vi "Add New Node In XML.vi"(6 "Data":string, 8 "error in (no error)":errorcluster, 9 "Tag Name":string, 10 "DOM document":refnum<k20>, 11 "XML Project in":refnum<class "XML Project.lvclass">) -> (0 "error out":errorcluster, 3 "XML Project out":refnum<class "XML Project.lvclass">)   [LabVIEW 2015, in "XML Project.lvclass"]
uses:
  XML Project.lvclass
  <resource>/objmgr/DOMUserDefRef.rc
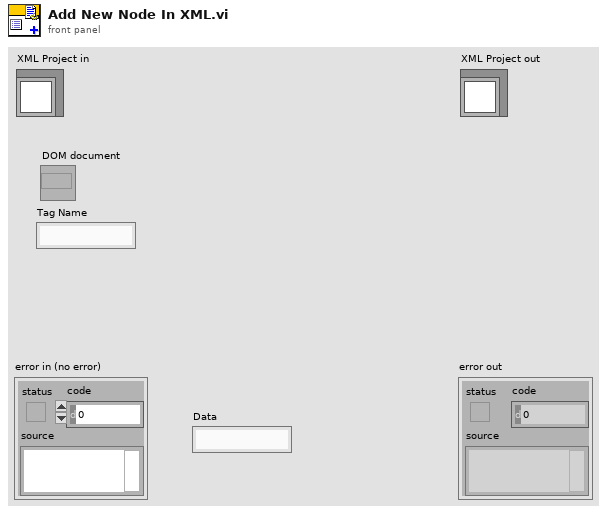
[diagram p1: front panel]
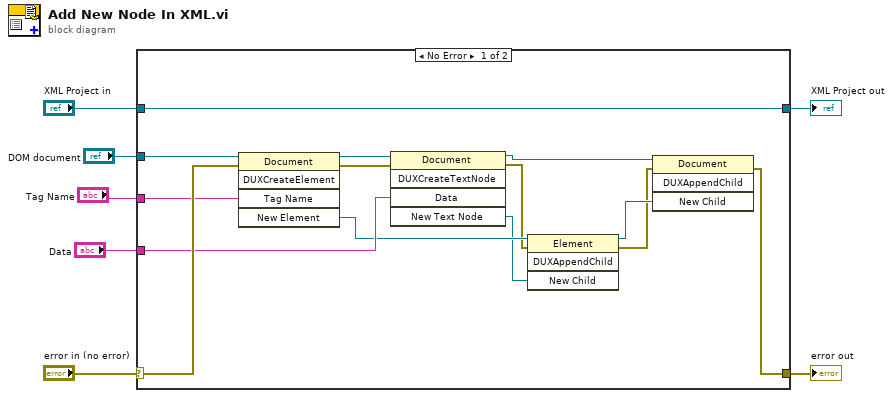
[diagram p0: block diagram]
diagram:
  n1 = case shown="No Error" "error in (no error)" {
    selector: "error in (no error)" -> [w19 w23]
    tunnel: [w8 w23] -> w6
    tunnel: [w21 w22] -> w4
    tunnel: "XML Project in" -> [w21 w22]
    tunnel: "DOM document" -> [w20 _]
    tunnel: "Tag Name" -> [w18 _]
    tunnel: "Data" -> [w15 _]
    frame No Error {
      n2 = invoke class="Document" method="DUXCreateElement"(reference=w20, error in=w19, "Tag Name"=w18) -> (reference out=w17:refnum<k20>, error out=w16:errorcluster, "New Element"=w14:refnum<k20>)  [unwired: 2 in, 2 out]
      n3 = invoke class="Document" method="DUXCreateTextNode"(reference=w17, error in=w16, "Data"=w15) -> (reference out=w11:refnum<k20>, error out=w12:errorcluster, "New Text Node"=w13:refnum<k20>)  [unwired: 2 in, 2 out]
      n4 = invoke class="Element" method="DUXAppendChild"(reference=w14, error in=w12, "New Child"=w13) -> (reference out=w10:refnum<k20>, error out=w9:errorcluster)  [unwired: 1 in, 2 out]
      n5 = invoke class="Document" method="DUXAppendChild"(reference=w11, error in=w9, "New Child"=w10) -> (error out=w8:errorcluster)  [unwired: 1 in, 3 out]
    }
    frame Error {
    }
  }
  "error out" <- w6
  "XML Project out" <- w4
